vi "Lighthouse Monitoring & Control System 9.vi"() -> ()   [LabVIEW 2012]
uses:
  <vilib>/DAQmx/read.llb/DAQmx Read (Counter DBL 1Chan 1Samp).vi
  <vilib>/DAQmx/write.llb/DAQmx Write (Analog DBL 1Chan 1Samp).vi
  <vilib>/DAQmx/write.llb/DAQmx Write (Digital U8 1Chan 1Samp).vi
  <vilib>/DAQmx/write.llb/DAQmx Write (Digital 1D Bool NChan 1Samp 1Line).vi
  <vilib>/DAQmx/read.llb/DAQmx Read (Analog DBL 1Chan 1Samp).vi
  <vilib>/DAQmx/create/channels.llb/DAQmx Create Channel (CI-Count Edges).vi
  <vilib>/DAQmx/create/channels.llb/DAQmx Create Channel (DO-Digital Output).vi
  <vilib>/DAQmx/create/channels.llb/DAQmx Create Channel (AI-Voltage-Basic).vi
  <vilib>/DAQmx/create/channels.llb/DAQmx Create Channel (AO-Voltage-Basic).vi
  <vilib>/DAQmx/miscellaneous.llb/DAQmx Fill In Error Info.vi
panel:
  out "Time:":string
  out "Date:":string
  out "Voltage:":dbl
  out "Slot Count:":dbl
  in  "Dignostic Mode":bool
  in  "?":bool
  out "Data to Write":u32=255 caption="Data to Write:" format="%x"
  out "Motor:":bool[](array[boolean])
  out "3":bool
  out "2":bool
  out "1":bool
  # "Lighthouse Monitoring & Control System"
  # "Normal Mode"
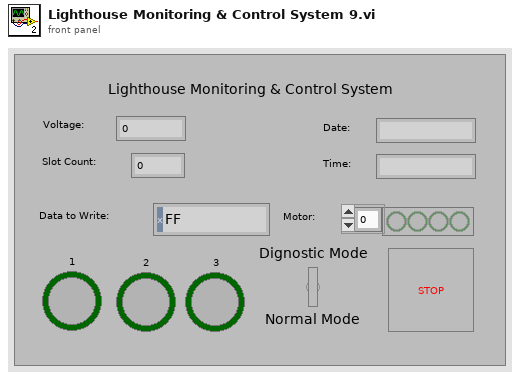
[diagram p1: front panel]
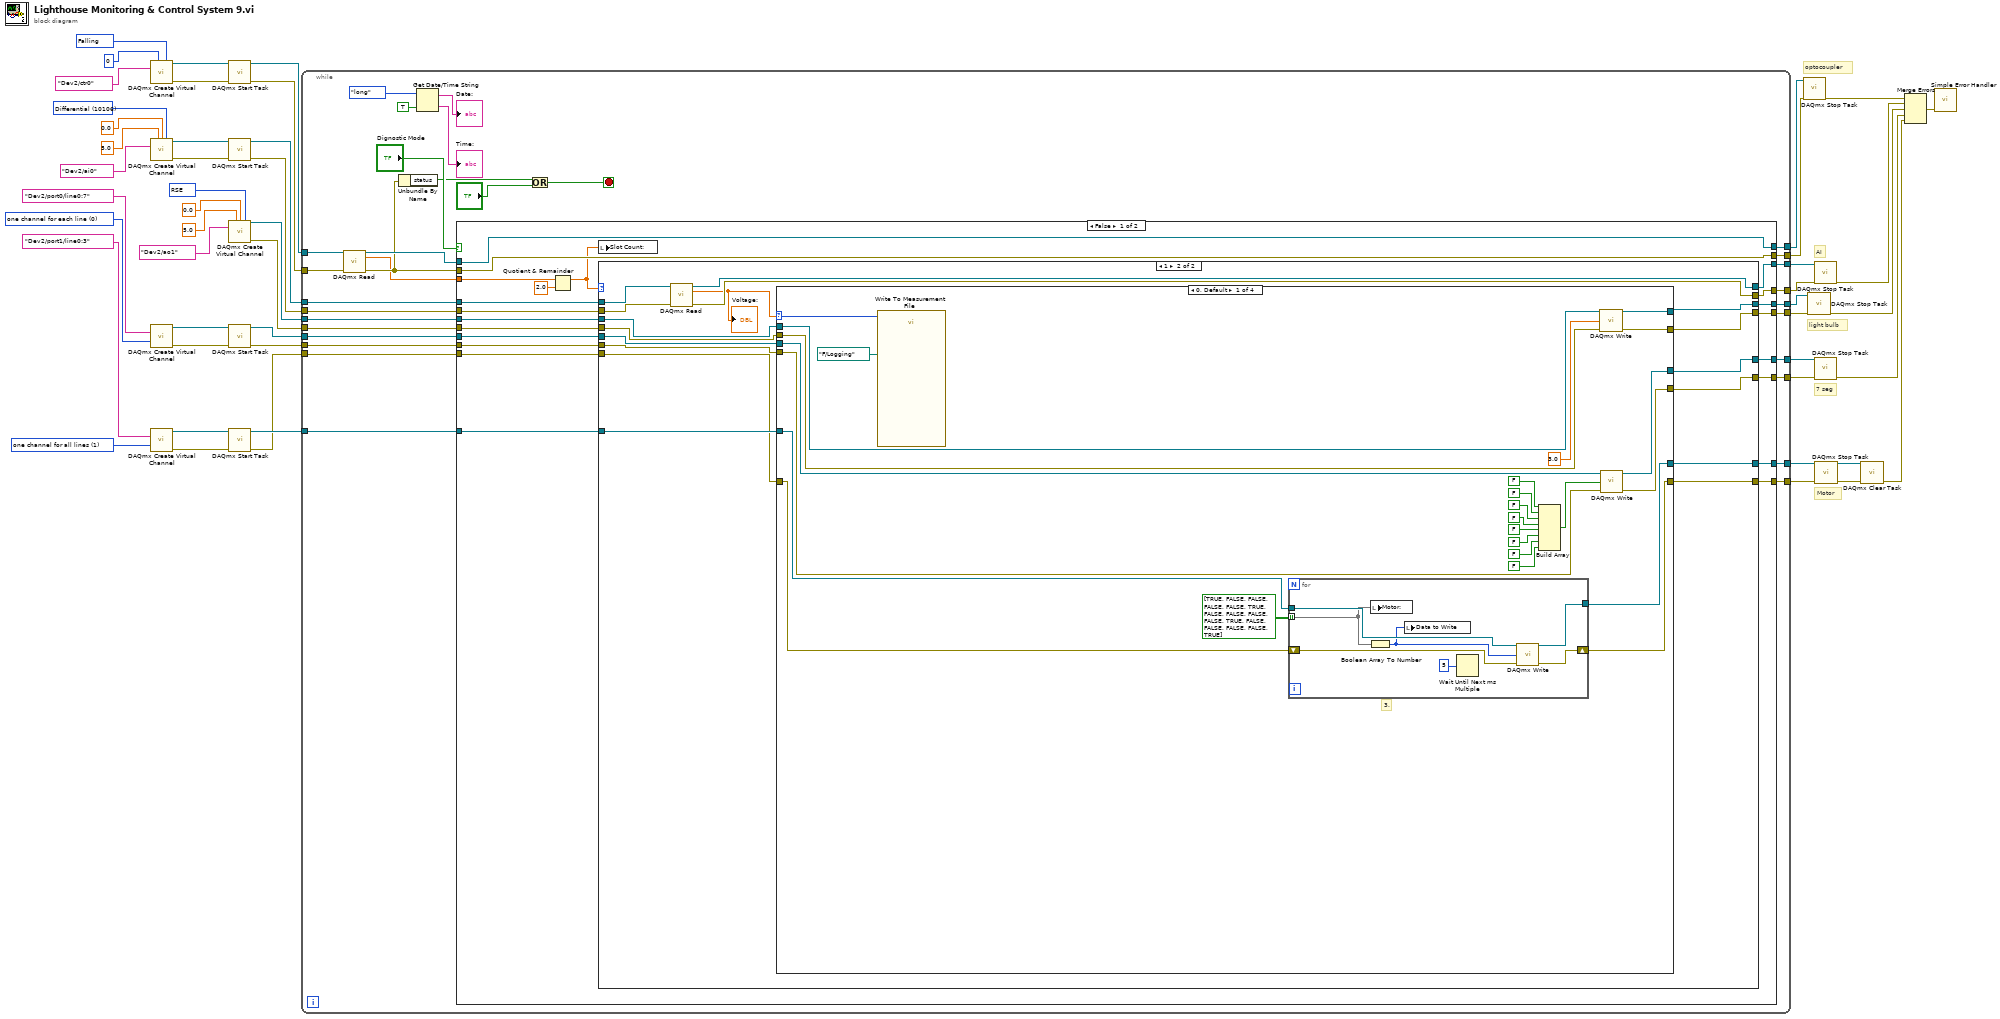
[diagram p0: block diagram]
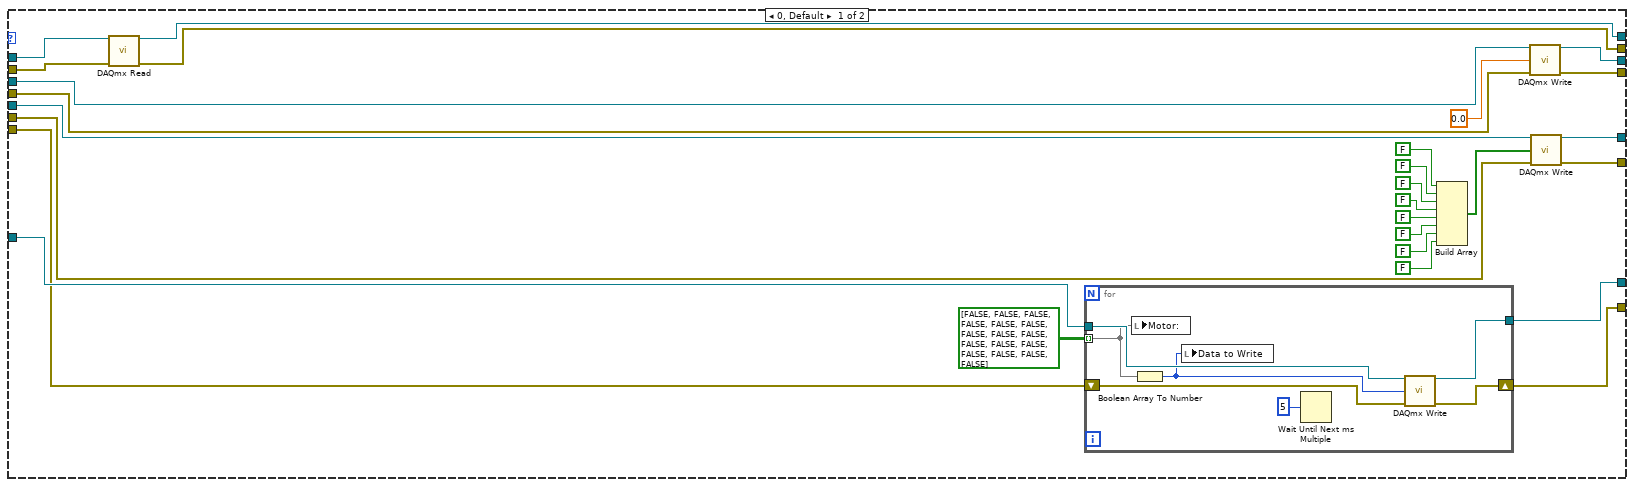
[diagram p2: hidden frame]
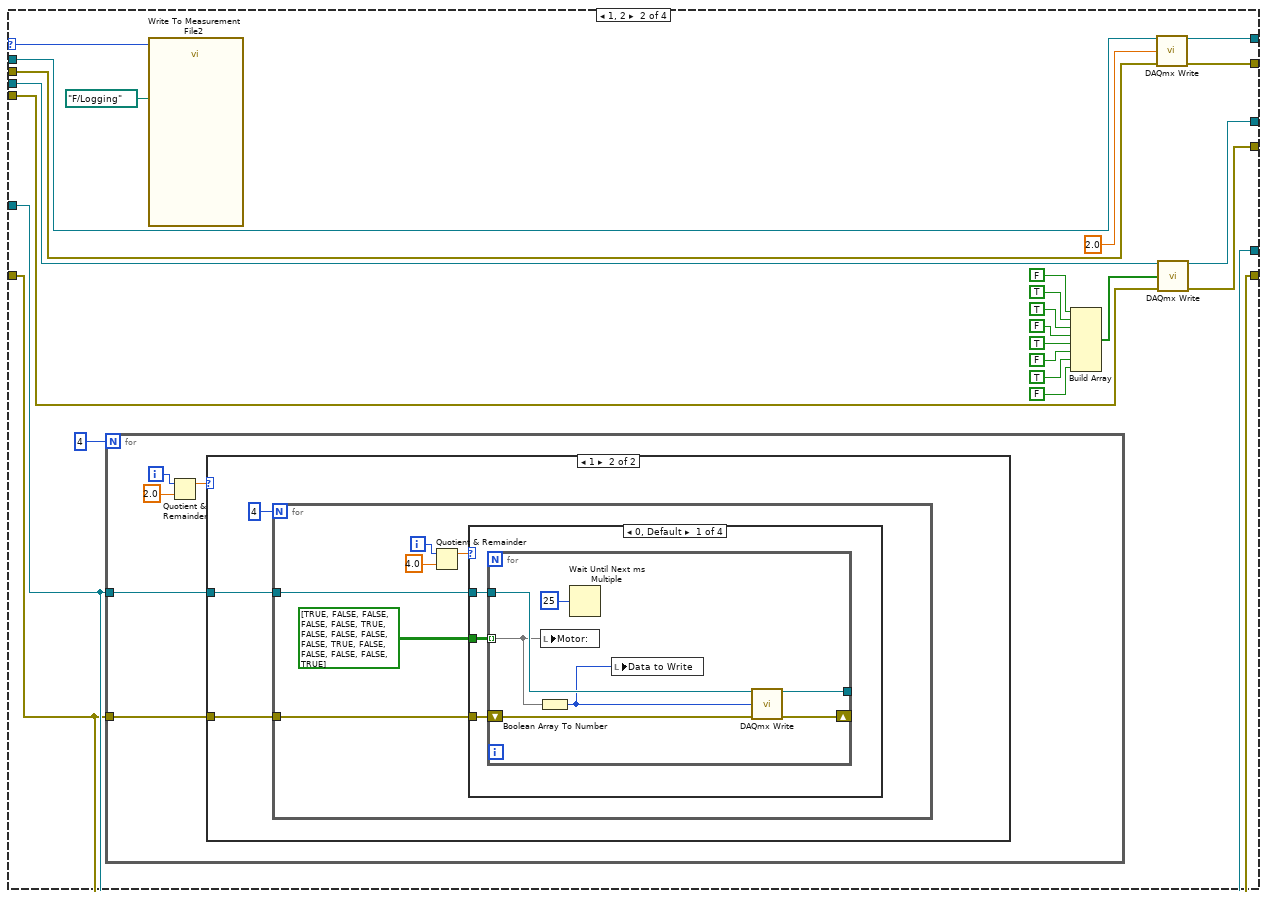
[diagram p3: hidden frame]
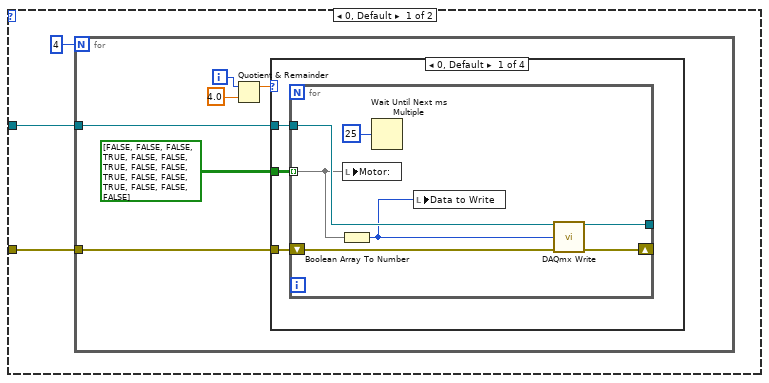
[diagram p4: hidden frame]
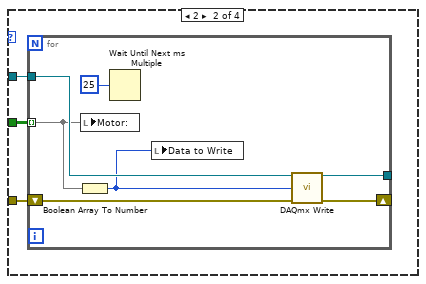
[diagram p5: hidden frame]
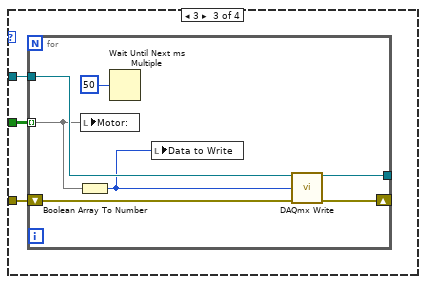
[diagram p6: hidden frame]
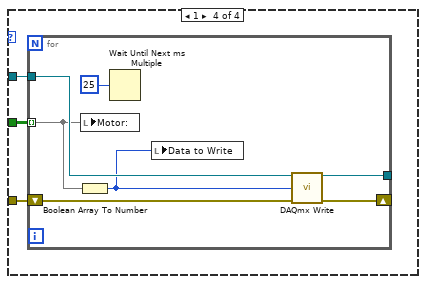
[diagram p7: hidden frame]
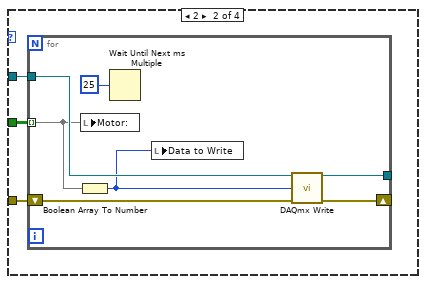
[diagram p8: hidden frame]
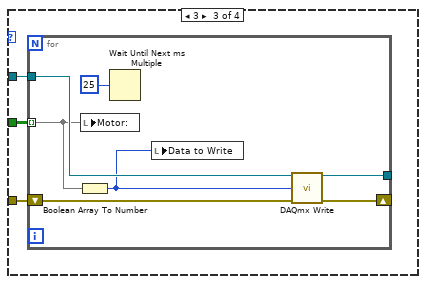
[diagram p9: hidden frame]
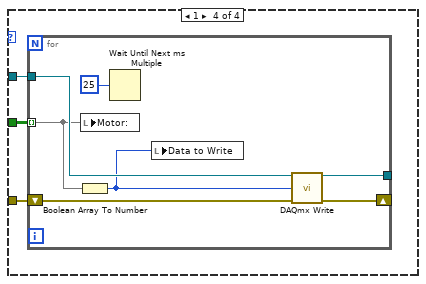
[diagram p10: hidden frame]
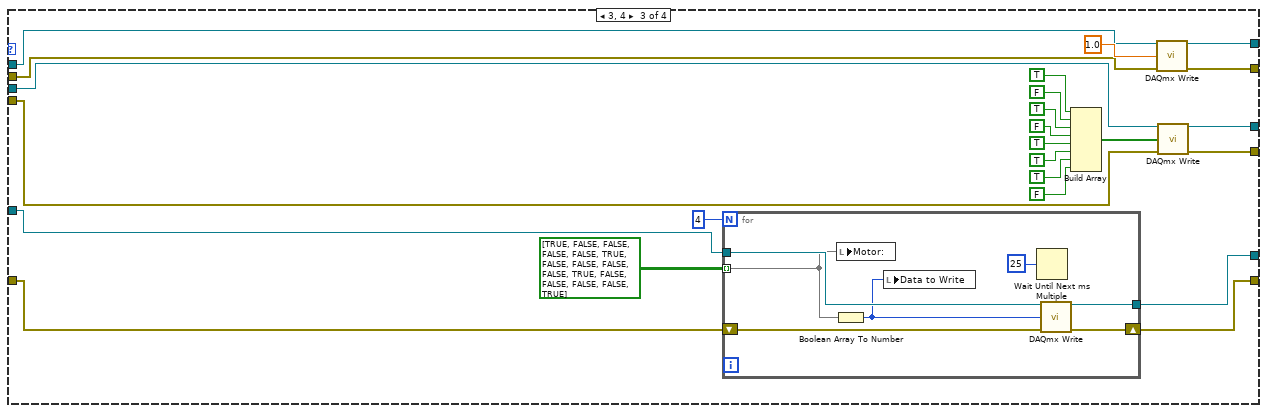
[diagram p11: hidden frame]
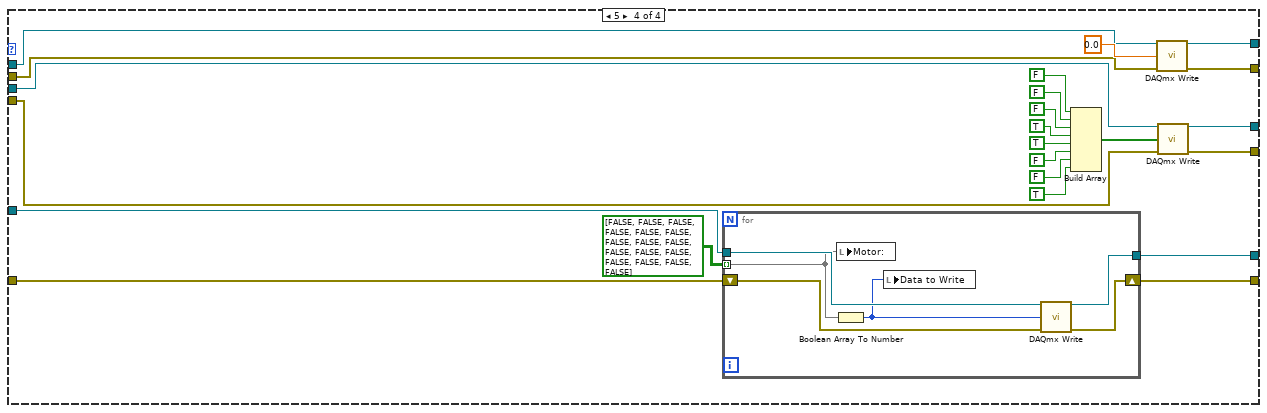
[diagram p12: hidden frame]
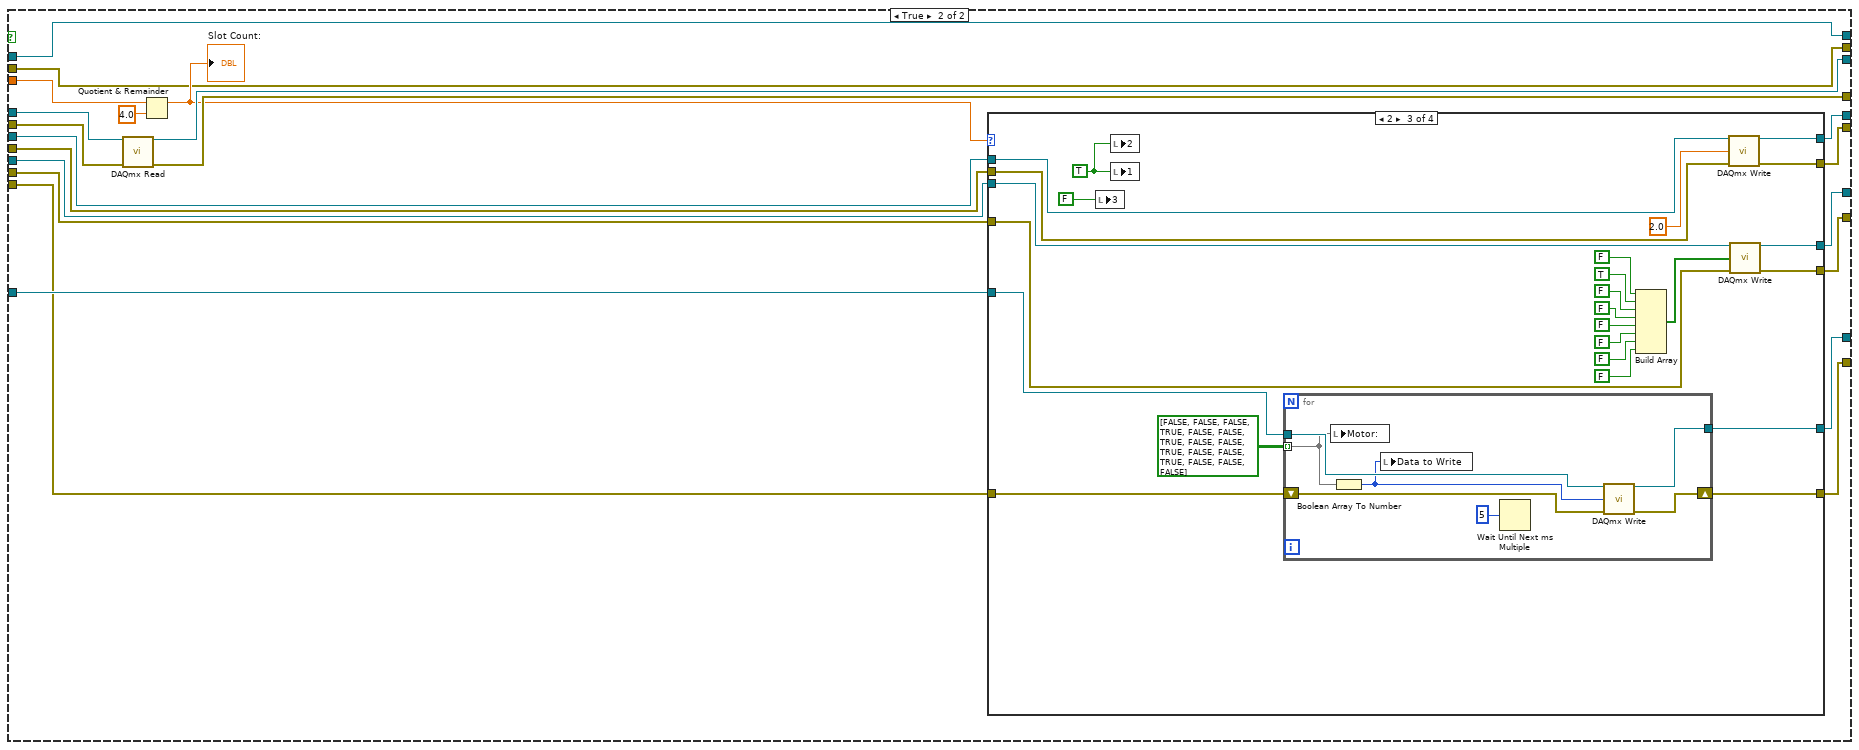
[diagram p13: hidden frame]
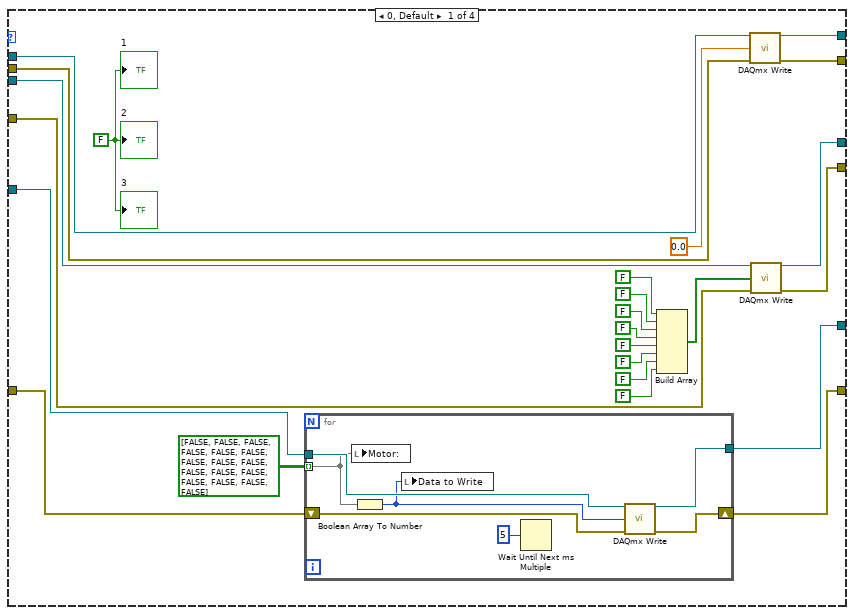
[diagram p14: hidden frame]
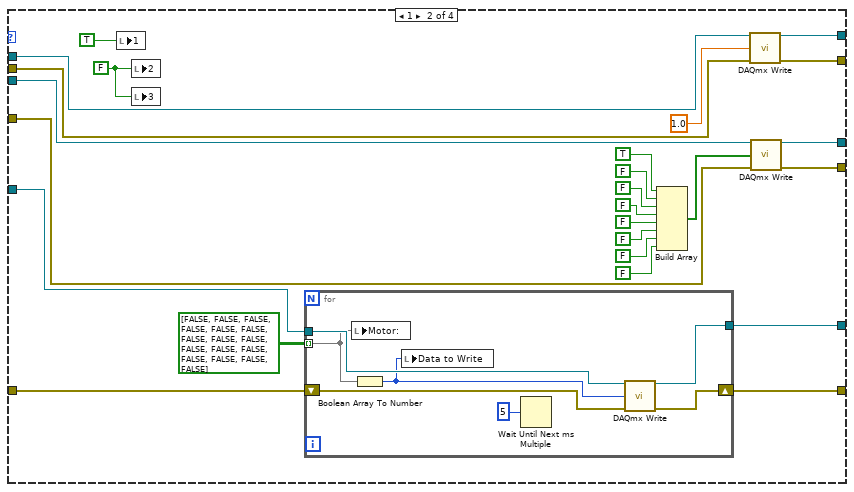
[diagram p15: hidden frame]
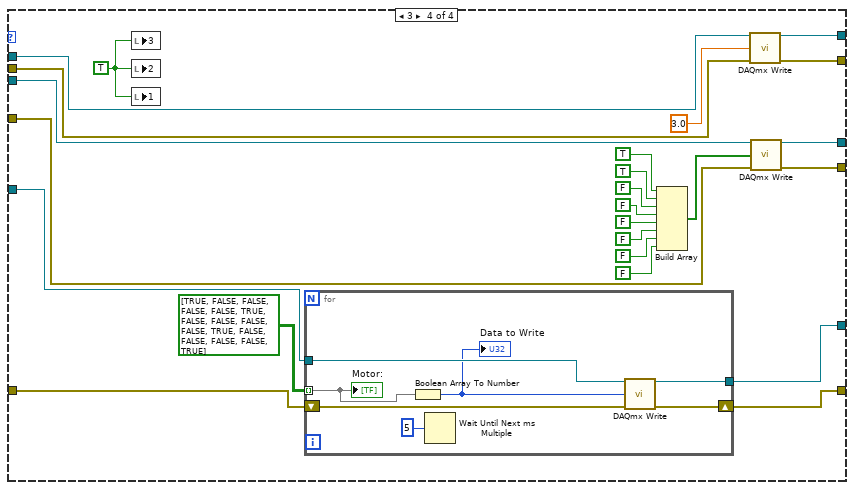
[diagram p16: hidden frame]
diagram:
  w24 = 10083 items=["Default"=-1, "RSE"=10083, "Differential"=10106, "Pseudodifferential"=12529] ("output terminal configuration")
  w32 = 10106 items=["default"=-1, "RSE"=10083, "NRSE"=10078, "Differential"=10106, "Pseudodifferential"=12529] ("input terminal configuration")
  w42 = 1 items=["one channel for each line", "one channel for all lines"] ("line grouping")
  w37 = 0 items=["one channel for each line", "one channel for all lines"] ("line grouping")
  w51 = 10171 items=["Rising"=10280, "Falling"=10171] ("edge")
  # "Motor"
  # "7 seg"
  # "AI"
  # "light bulb"
  # "optocoupler"
  n1 = call-poly <vilib>:"DAQmx Create Virtual Channel.vi"("initial count"=u32 0, "edge"=w51, "counter"=tag "Dev2/ctr0") -> ("task out"=w50:refnum<k21>, "error out"=w49:errorcluster)  [unwired: 11 in]
  n2 = call-poly <vilib>:"DAQmx Create Virtual Channel.vi"("maximum value"=5.0, "minimum value"=0.0, "input terminal configuration"=w32, "physical channels"=tag "Dev2/ai0") -> ("task out"=w30:refnum<k21>, "error out"=w31:errorcluster)  [unwired: 10 in]
  n3 = call-poly <vilib>:"DAQmx Create Virtual Channel.vi"("lines"=tag "Dev2/port0/line0:7", "line grouping"=w37) -> ("task out"=w44:refnum<k21>, "error out"=w43:errorcluster)  [unwired: 12 in]
  n4 = call-poly <vilib>:"DAQmx Create Virtual Channel.vi"("lines"=tag "Dev2/port1/line0:3", "line grouping"=w42) -> ("task out"=w41:refnum<k21>, "error out"=w40:errorcluster)  [unwired: 12 in]
  n5 = call <vilib>:"DAQmx Start Task.vi"("task/channels in"=w50, "error in"=w49) -> ("task out"=w46:refnum<k21>, "error out"=w45:errorcluster)  [unwired: 12 in]
  n6 = call <vilib>:"DAQmx Start Task.vi"("task/channels in"=w30, "error in"=w31) -> ("task out"=w26:refnum<k21>, "error out"=w25:errorcluster)  [unwired: 12 in]
  n7 = call-poly <vilib>:"DAQmx Create Virtual Channel.vi"("maximum value"=5.0, "minimum value"=0.0, "output terminal configuration"=w24, "physical channels"=tag "Dev2/ao1") -> ("task out"=w20:refnum<k21>, "error out"=w19:errorcluster)  [unwired: 10 in]
  n8 = call <vilib>:"DAQmx Start Task.vi"("task/channels in"=w44, "error in"=w43) -> ("task out"=w36:refnum<k21>, "error out"=w35:errorcluster)  [unwired: 12 in]
  n9 = call <vilib>:"DAQmx Start Task.vi"("task/channels in"=w41, "error in"=w40) -> ("task out"=w34:refnum<k21>, "error out"=w33:errorcluster)  [unwired: 12 in]
  n10 = while {
    tunnel: w46 -> [w81]
    tunnel: w45 -> [w80]
    tunnel: w36 -> [w79]
    tunnel: w35 -> [w78]
    tunnel: w34 -> [w77]
    tunnel: w33 -> [w76]
    tunnel: w26 -> [w74]
    tunnel: w25 -> [w73]
    tunnel: w20 -> [w72]
    tunnel: w19 -> [w71]
    tunnel: [w65] -> w10
    tunnel: [w64] -> w9
    tunnel: [w63] -> w8
    tunnel: [w62] -> w7
    tunnel: [w61] -> w6
    tunnel: [w60] -> w5
    tunnel: [w59] -> w4
    tunnel: [w58] -> w3
    tunnel: [w57] -> w2
    tunnel: [w56] -> w1
    stop <- w66 stop-if-true
    n11 = call-poly <vilib>:"DAQmx Read.vi"("task/channels in"=w81, "error in"=w80) -> ("task out"=w69:refnum<k21>, "data"=w67:dbl, "error out"=w68:errorcluster)  [unwired: 11 in]
    n12 = Unbundle By Name(w68) -> ("status"=w75:bool)
    n13 = Get Date/Time String(date format (0)=enum16{"short", "long", "abbreviated"}."long", want seconds? (F)=TRUE) -> (date string=→"Date:":string, time string=→"Time:":string)  [unwired: 1 in]
    n14 = case shown="False" "Dignostic Mode" {
      tunnel: w79 -> [w91 w393]
      tunnel: w78 -> [w90 w392]
      tunnel: w77 -> [w89 w391]
      tunnel: w76 -> [w88 w390]
      tunnel: [w87 w389] -> w59
      tunnel: [w86 w388] -> w58
      tunnel: w74 -> [w101 w385]
      tunnel: w73 -> [w100 w384]
      tunnel: w72 -> [w85 w387]
      tunnel: w71 -> [w84 w386]
      tunnel: [w99 w383] -> w57
      tunnel: [w98 w382] -> w56
      tunnel: [w97 w381] -> w63
      tunnel: [w96 w380] -> w62
      tunnel: [w93 w379] -> w60
      tunnel: [w92 w378] -> w61
      tunnel: w69 -> [w95 w374]
      tunnel: w68 -> [w94 w373]
      tunnel: w67 -> [w102 w376]
      tunnel: [w95 w374] -> w65
      tunnel: [w94 w373] -> w64
      frame False {
        n15 = Quotient & Remainder(x=w102, y=2.0) -> (x-y*floor(x/y)=w83:dbl)  [unwired: 1 out]
        n16 = local write "Slot Count:"(w83) -> ()
        n17 = case shown="1" w83 {
          tunnel: w101 -> [w129 w154]
          tunnel: w100 -> [w128 w153]
          tunnel: [w125 w152] -> w97
          tunnel: [w126 w151] -> w96
          tunnel: [w127 w150] -> w98
          tunnel: [w122 w149] -> w93
          tunnel: [w123 w148] -> w92
          tunnel: [w124 w147] -> w99
          tunnel: [w110 w145] -> w86
          tunnel: [w111 w146] -> w87
          tunnel: w91 -> [w109 w139]
          tunnel: w90 -> [w108 w138]
          tunnel: w89 -> [w107 w141]
          tunnel: w88 -> [w106 w140]
          tunnel: w85 -> [w105 w143]
          tunnel: w84 -> [w104 w142]
          frame 0, Default {
            n18 = call-poly <vilib>:"DAQmx Read.vi"("task/channels in"=w129, "error in"=w128) -> ("task out"=w124:refnum<k21>, "error out"=w127:errorcluster)  [unwired: 11 in, 1 out]
            n19 = for {
              tunnel: [w136] -> w111
              shift-right: [w134] -> w110
              shift-left: w106 -> [w137]
              tunnel: bool[][] [[FALSE, FALSE, FALSE, FALSE], [FALSE, FALSE, FALSE, FALSE], [FALSE, FALSE, FALSE, FALSE], [FALSE, FALSE, FALSE, FALSE]] -> [w131] mode=indexing
              tunnel: w107 -> [w133]
              n20 = local write "Motor:"(w131) -> ()
              n21 = Boolean Array To Number(Boolean array=w131) -> (number=w132:u32)
              n22 = local write "Data to Write"(w132) -> ()
              n23 = Wait Until Next ms Multiple(millisecond multiple=5) -> ()  [unwired: 1 out]
              n24 = call-poly <vilib>:"DAQmx Write.vi"("task/channels in"=w133, "data"=w132, "error in"=w137) -> ("task out"=w136:refnum<k21>, "error out"=w134:errorcluster)  [unwired: 10 in, 1 out]
            }
            n25 = Build Array(FALSE, FALSE, FALSE, FALSE, FALSE, FALSE, FALSE, FALSE) -> (w113:bool[])
            n26 = call-poly <vilib>:"DAQmx Write.vi"("task/channels in"=w105, "data"=0.0, "error in"=w104) -> ("task out"=w125:refnum<k21>, "error out"=w126:errorcluster)  [unwired: 10 in, 1 out]
            n27 = call-poly <vilib>:"DAQmx Write.vi"("task/channels in"=w109, "data"=w113, "error in"=w108) -> ("task out"=w123:refnum<k21>, "error out"=w122:errorcluster)  [unwired: 10 in, 1 out]
          }
          frame 1 {
            n28 = call-poly <vilib>:"DAQmx Read.vi"("task/channels in"=w154, "error in"=w153) -> ("task out"=w147:refnum<k21>, "data"=w144:dbl, "error out"=w150:errorcluster)  [unwired: 11 in]
            "Voltage:" <- w144
            n29 = case shown="0, Default" w144 {
              selector: w144 -> [w161 w194 _ _]
              tunnel: [w169 w199 w326 w356] -> w152
              tunnel: [w168 w198 w325 w355] -> w151
              tunnel: [w167 w197 w324 w354] -> w148
              tunnel: [w166 w196 w323 w353] -> w149
              tunnel: [w165 w188 w321 w351] -> w146
              tunnel: [w164 w187 w320 w350] -> w145
              tunnel: w143 -> [w160 w193 w319 w349]
              tunnel: w142 -> [w159 w192 w318 w348]
              tunnel: w141 -> [w158 w188 w315 w345]
              tunnel: w140 -> [w155 w187 w314 w344]
              tunnel: w139 -> [w157 w191 w317 w347]
              tunnel: w138 -> [w156 w190 w316 w346]
              frame 0, Default {
                # "3."
                n30 = call "Write To Measurement File"("Signals"=w161, "Filename"=path "F:/Logging") -> ()  [unwired: 15 in, 3 out]
                n31 = for {
                  tunnel: [w185] -> w165
                  shift-right: [w184] -> w164
                  shift-left: w155 -> [w186]
                  tunnel: bool[][] [[TRUE, FALSE, FALSE, FALSE], [FALSE, TRUE, FALSE, FALSE], [FALSE, FALSE, TRUE, FALSE], [FALSE, FALSE, FALSE, TRUE]] -> [w180] mode=indexing
                  tunnel: w158 -> [w182]
                  n32 = Boolean Array To Number(Boolean array=w180) -> (number=w181:u32)
                  n33 = local write "Motor:"(w180) -> ()
                  n34 = local write "Data to Write"(w181) -> ()
                  n35 = Wait Until Next ms Multiple(millisecond multiple=u32 5) -> ()  [unwired: 1 out]
                  n36 = call-poly <vilib>:"DAQmx Write.vi"("task/channels in"=w182, "data"=w181, "error in"=w186) -> ("task out"=w185:refnum<k21>, "error out"=w184:errorcluster)  [unwired: 10 in, 1 out]
                }
                n37 = Build Array(FALSE, FALSE, FALSE, FALSE, FALSE, FALSE, FALSE, FALSE) -> (w170:bool[])
                n38 = call-poly <vilib>:"DAQmx Write.vi"("task/channels in"=w160, "data"=3.0, "error in"=w159) -> ("task out"=w169:refnum<k21>, "error out"=w168:errorcluster)  [unwired: 10 in, 1 out]
                n39 = call-poly <vilib>:"DAQmx Write.vi"("task/channels in"=w157, "data"=w170, "error in"=w156) -> ("task out"=w167:refnum<k21>, "error out"=w166:errorcluster)  [unwired: 10 in, 1 out]
              }
              frame 1, 2 {
                n40 = for {
                  N: 4 -> [_]
                  tunnel: w188 -> [w214]
                  tunnel: w187 -> [w213]
                  i -> [w211]
                  n41 = Quotient & Remainder(x=w211, y=2.0) -> (x-y*floor(x/y)=w210:dbl)  [unwired: 1 out]
                  n42 = case shown="1" w210 {
                    tunnel: w214 -> [w217 w266]
                    tunnel: w213 -> [w216 w265]
                    frame 0, Default {
                      n43 = for {
                        N: 4 -> [_]
                        tunnel: w217 -> [w223]
                        tunnel: w216 -> [w222]
                        i -> [w219]
                        n44 = Quotient & Remainder(x=w219, y=4.0) -> (x-y*floor(x/y)=w218:dbl)  [unwired: 1 out]
                        n45 = case shown="0, Default" w218 {
                          tunnel: w223 -> [w226 w236 w245 w256]
                          tunnel: w222 -> [w224 w235 w246 w255]
                          tunnel: bool[][] [[FALSE, FALSE, FALSE, TRUE], [FALSE, FALSE, TRUE, FALSE], [FALSE, TRUE, FALSE, FALSE], [TRUE, FALSE, FALSE, FALSE]] -> [w225 w234 w244 w254]
                          frame 0, Default {
                            n46 = for {
                              tunnel: [w232] -> _
                              shift-right: [w231] -> _
                              shift-left: w224 -> [w233]
                              tunnel: w225 -> [w227] mode=indexing
                              tunnel: w226 -> [w229]
                              n47 = Boolean Array To Number(Boolean array=w227) -> (number=w228:u32)
                              n48 = local write "Motor:"(w227) -> ()
                              n49 = Wait Until Next ms Multiple(millisecond multiple=u32 25) -> ()  [unwired: 1 out]
                              n50 = local write "Data to Write"(w228) -> ()
                              n51 = call-poly <vilib>:"DAQmx Write.vi"("task/channels in"=w229, "data"=w228, "error in"=w233) -> ("task out"=w232:refnum<k21>, "error out"=w231:errorcluster)  [unwired: 10 in, 1 out]
                            }
                          }
                          frame 2 {
                            n52 = for {
                              tunnel: [w242] -> _
                              shift-right: [w241] -> _
                              shift-left: w235 -> [w243]
                              tunnel: w234 -> [w237] mode=indexing
                              tunnel: w236 -> [w239]
                              n53 = Boolean Array To Number(Boolean array=w237) -> (number=w238:u32)
                              n54 = local write "Motor:"(w237) -> ()
                              n55 = Wait Until Next ms Multiple(millisecond multiple=u32 25) -> ()  [unwired: 1 out]
                              n56 = local write "Data to Write"(w238) -> ()
                              n57 = call-poly <vilib>:"DAQmx Write.vi"("task/channels in"=w239, "data"=w238, "error in"=w243) -> ("task out"=w242:refnum<k21>, "error out"=w241:errorcluster)  [unwired: 10 in, 1 out]
                            }
                          }
                          frame 3 {
                            n58 = for {
                              tunnel: [w252] -> _
                              shift-right: [w251] -> _
                              shift-left: w246 -> [w253]
                              tunnel: w244 -> [w248] mode=indexing
                              tunnel: w245 -> [w249]
                              n59 = Boolean Array To Number(Boolean array=w248) -> (number=w247:u32)
                              n60 = local write "Motor:"(w248) -> ()
                              n61 = Wait Until Next ms Multiple(millisecond multiple=u32 50) -> ()  [unwired: 1 out]
                              n62 = local write "Data to Write"(w247) -> ()
                              n63 = call-poly <vilib>:"DAQmx Write.vi"("task/channels in"=w249, "data"=w247, "error in"=w253) -> ("task out"=w252:refnum<k21>, "error out"=w251:errorcluster)  [unwired: 10 in, 1 out]
                            }
                          }
                          frame 1 {
                            n64 = for {
                              tunnel: [w262] -> _
                              shift-right: [w261] -> _
                              shift-left: w255 -> [w263]
                              tunnel: w254 -> [w258] mode=indexing
                              tunnel: w256 -> [w259]
                              n65 = Boolean Array To Number(Boolean array=w258) -> (number=w257:u32)
                              n66 = local write "Motor:"(w258) -> ()
                              n67 = Wait Until Next ms Multiple(millisecond multiple=u32 25) -> ()  [unwired: 1 out]
                              n68 = local write "Data to Write"(w257) -> ()
                              n69 = call-poly <vilib>:"DAQmx Write.vi"("task/channels in"=w259, "data"=w257, "error in"=w263) -> ("task out"=w262:refnum<k21>, "error out"=w261:errorcluster)  [unwired: 10 in, 1 out]
                            }
                          }
                        }
                      }
                    }
                    frame 1 {
                      n70 = for {
                        N: 4 -> [_]
                        tunnel: w266 -> [w272]
                        tunnel: w265 -> [w271]
                        i -> [w270]
                        n71 = Quotient & Remainder(x=w270, y=4.0) -> (x-y*floor(x/y)=w268:dbl)  [unwired: 1 out]
                        n72 = case shown="0, Default" w268 {
                          tunnel: w272 -> [w275 w285 w294 w305]
                          tunnel: w271 -> [w274 w284 w295 w304]
                          tunnel: bool[][] [[TRUE, FALSE, FALSE, FALSE], [FALSE, TRUE, FALSE, FALSE], [FALSE, FALSE, TRUE, FALSE], [FALSE, FALSE, FALSE, TRUE]] -> [w273 w283 w293 w303]
                          frame 0, Default {
                            n73 = for {
                              tunnel: [w281] -> _
                              shift-right: [w280] -> _
                              shift-left: w274 -> [w282]
                              tunnel: w273 -> [w277] mode=indexing
                              tunnel: w275 -> [w278]
                              n74 = Boolean Array To Number(Boolean array=w277) -> (number=w276:u32)
                              n75 = local write "Motor:"(w277) -> ()
                              n76 = Wait Until Next ms Multiple(millisecond multiple=u32 25) -> ()  [unwired: 1 out]
                              n77 = local write "Data to Write"(w276) -> ()
                              n78 = call-poly <vilib>:"DAQmx Write.vi"("task/channels in"=w278, "data"=w276, "error in"=w282) -> ("task out"=w281:refnum<k21>, "error out"=w280:errorcluster)  [unwired: 10 in, 1 out]
                            }
                          }
                          frame 2 {
                            n79 = for {
                              tunnel: [w291] -> _
                              shift-right: [w290] -> _
                              shift-left: w284 -> [w292]
                              tunnel: w283 -> [w286] mode=indexing
                              tunnel: w285 -> [w288]
                              n80 = Boolean Array To Number(Boolean array=w286) -> (number=w287:u32)
                              n81 = local write "Motor:"(w286) -> ()
                              n82 = Wait Until Next ms Multiple(millisecond multiple=u32 25) -> ()  [unwired: 1 out]
                              n83 = local write "Data to Write"(w287) -> ()
                              n84 = call-poly <vilib>:"DAQmx Write.vi"("task/channels in"=w288, "data"=w287, "error in"=w292) -> ("task out"=w291:refnum<k21>, "error out"=w290:errorcluster)  [unwired: 10 in, 1 out]
                            }
                          }
                          frame 3 {
                            n85 = for {
                              tunnel: [w301] -> _
                              shift-right: [w300] -> _
                              shift-left: w295 -> [w302]
                              tunnel: w293 -> [w297] mode=indexing
                              tunnel: w294 -> [w298]
                              n86 = Boolean Array To Number(Boolean array=w297) -> (number=w296:u32)
                              n87 = local write "Motor:"(w297) -> ()
                              n88 = Wait Until Next ms Multiple(millisecond multiple=u32 25) -> ()  [unwired: 1 out]
                              n89 = local write "Data to Write"(w296) -> ()
                              n90 = call-poly <vilib>:"DAQmx Write.vi"("task/channels in"=w298, "data"=w296, "error in"=w302) -> ("task out"=w301:refnum<k21>, "error out"=w300:errorcluster)  [unwired: 10 in, 1 out]
                            }
                          }
                          frame 1 {
                            n91 = for {
                              tunnel: [w311] -> _
                              shift-right: [w310] -> _
                              shift-left: w304 -> [w312]
                              tunnel: w303 -> [w307] mode=indexing
                              tunnel: w305 -> [w308]
                              n92 = Boolean Array To Number(Boolean array=w307) -> (number=w306:u32)
                              n93 = local write "Motor:"(w307) -> ()
                              n94 = Wait Until Next ms Multiple(millisecond multiple=u32 25) -> ()  [unwired: 1 out]
                              n95 = local write "Data to Write"(w306) -> ()
                              n96 = call-poly <vilib>:"DAQmx Write.vi"("task/channels in"=w308, "data"=w306, "error in"=w312) -> ("task out"=w311:refnum<k21>, "error out"=w310:errorcluster)  [unwired: 10 in, 1 out]
                            }
                          }
                        }
                      }
                    }
                  }
                }
                n97 = call "Write To Measurement File2"("Signals"=w194, "Filename"=path "F:/Logging") -> ()  [unwired: 15 in, 3 out]
                n98 = Build Array(FALSE, TRUE, TRUE, FALSE, TRUE, FALSE, TRUE, FALSE) -> (w200:bool[])
                n99 = call-poly <vilib>:"DAQmx Write.vi"("task/channels in"=w193, "data"=2.0, "error in"=w192) -> ("task out"=w199:refnum<k21>, "error out"=w198:errorcluster)  [unwired: 10 in, 1 out]
                n100 = call-poly <vilib>:"DAQmx Write.vi"("task/channels in"=w191, "data"=w200, "error in"=w190) -> ("task out"=w197:refnum<k21>, "error out"=w196:errorcluster)  [unwired: 10 in, 1 out]
              }
              frame 3, 4 {
                n101 = for {
                  N: 4 -> [_]
                  tunnel: [w342] -> w321
                  shift-right: [w341] -> w320
                  shift-left: w314 -> [w343]
                  tunnel: bool[][] [[TRUE, FALSE, FALSE, FALSE], [FALSE, TRUE, FALSE, FALSE], [FALSE, FALSE, TRUE, FALSE], [FALSE, FALSE, FALSE, TRUE]] -> [w338] mode=indexing
                  tunnel: w315 -> [w340]
                  n102 = Boolean Array To Number(Boolean array=w338) -> (number=w339:u32)
                  n103 = local write "Motor:"(w338) -> ()
                  n104 = local write "Data to Write"(w339) -> ()
                  n105 = Wait Until Next ms Multiple(millisecond multiple=u32 25) -> ()  [unwired: 1 out]
                  n106 = call-poly <vilib>:"DAQmx Write.vi"("task/channels in"=w340, "data"=w339, "error in"=w343) -> ("task out"=w342:refnum<k21>, "error out"=w341:errorcluster)  [unwired: 10 in, 1 out]
                }
                n107 = Build Array(TRUE, FALSE, TRUE, FALSE, TRUE, TRUE, TRUE, FALSE) -> (w327:bool[])
                n108 = call-poly <vilib>:"DAQmx Write.vi"("task/channels in"=w319, "data"=1.0, "error in"=w318) -> ("task out"=w326:refnum<k21>, "error out"=w325:errorcluster)  [unwired: 10 in, 1 out]
                n109 = call-poly <vilib>:"DAQmx Write.vi"("task/channels in"=w317, "data"=w327, "error in"=w316) -> ("task out"=w324:refnum<k21>, "error out"=w323:errorcluster)  [unwired: 10 in, 1 out]
              }
              frame 5 {
                n110 = for {
                  tunnel: [w371] -> w351
                  shift-right: [w370] -> w350
                  shift-left: w344 -> [w372]
                  tunnel: bool[][] [[FALSE, FALSE, FALSE, FALSE], [FALSE, FALSE, FALSE, FALSE], [FALSE, FALSE, FALSE, FALSE], [FALSE, FALSE, FALSE, FALSE]] -> [w367] mode=indexing
                  tunnel: w345 -> [w369]
                  n111 = Boolean Array To Number(Boolean array=w367) -> (number=w368:u32)
                  n112 = local write "Motor:"(w367) -> ()
                  n113 = local write "Data to Write"(w368) -> ()
                  n114 = call-poly <vilib>:"DAQmx Write.vi"("task/channels in"=w369, "data"=w368, "error in"=w372) -> ("task out"=w371:refnum<k21>, "error out"=w370:errorcluster)  [unwired: 10 in, 1 out]
                }
                n115 = Build Array(FALSE, FALSE, FALSE, TRUE, TRUE, FALSE, FALSE, TRUE) -> (w357:bool[])
                n116 = call-poly <vilib>:"DAQmx Write.vi"("task/channels in"=w349, "data"=0.0, "error in"=w348) -> ("task out"=w356:refnum<k21>, "error out"=w355:errorcluster)  [unwired: 10 in, 1 out]
                n117 = call-poly <vilib>:"DAQmx Write.vi"("task/channels in"=w347, "data"=w357, "error in"=w346) -> ("task out"=w354:refnum<k21>, "error out"=w353:errorcluster)  [unwired: 10 in, 1 out]
              }
            }
          }
        }
      }
      frame True {
        n118 = call-poly <vilib>:"DAQmx Read.vi"("task/channels in"=w385, "error in"=w384) -> ("task out"=w383:refnum<k21>, "error out"=w382:errorcluster)  [unwired: 11 in, 1 out]
        n119 = Quotient & Remainder(x=w376, y=4.0) -> (x-y*floor(x/y)=w375:dbl)  [unwired: 1 out]
        "Slot Count:" <- w375
        n120 = case shown="2" w375 {
          tunnel: w393 -> [w405 w433 w465 w496]
          tunnel: w392 -> [w404 w432 w466 w497]
          tunnel: w391 -> [w417 w431 w462 w494]
          tunnel: w390 -> [w416 w430 w463 w493]
          tunnel: [w415 w429 w461 w492] -> w389
          tunnel: [w414 w428 w460 w491] -> w388
          tunnel: w387 -> [w402 w444 w478 w509]
          tunnel: w386 -> [w401 w443 w477 w508]
          tunnel: [w400 w446 w480 w511] -> w381
          tunnel: [w399 w445 w479 w510] -> w380
          tunnel: [w396 w426 w458 w490] -> w378
          tunnel: [w395 w425 w457 w489] -> w379
          frame 0, Default {
            w397 = FALSE
            n121 = for {
              tunnel: [w423] -> w415
              shift-right: [w421] -> w414
              shift-left: w416 -> [w424]
              tunnel: w417 -> [w420]
              tunnel: bool[][] [[FALSE, FALSE, FALSE, FALSE], [FALSE, FALSE, FALSE, FALSE], [FALSE, FALSE, FALSE, FALSE], [FALSE, FALSE, FALSE, FALSE]] -> [w418] mode=indexing
              n122 = local write "Motor:"(w418) -> ()
              n123 = Boolean Array To Number(Boolean array=w418) -> (number=w419:u32)
              n124 = local write "Data to Write"(w419) -> ()
              n125 = Wait Until Next ms Multiple(millisecond multiple=5) -> ()  [unwired: 1 out]
              n126 = call-poly <vilib>:"DAQmx Write.vi"("task/channels in"=w420, "data"=w419, "error in"=w424) -> ("task out"=w423:refnum<k21>, "error out"=w421:errorcluster)  [unwired: 10 in, 1 out]
            }
            n127 = Build Array(FALSE, FALSE, FALSE, FALSE, FALSE, FALSE, FALSE, FALSE) -> (w406:bool[])
            n128 = call-poly <vilib>:"DAQmx Write.vi"("task/channels in"=w402, "data"=0.0, "error in"=w401) -> ("task out"=w400:refnum<k21>, "error out"=w399:errorcluster)  [unwired: 10 in, 1 out]
            n129 = call-poly <vilib>:"DAQmx Write.vi"("task/channels in"=w405, "data"=w406, "error in"=w404) -> ("task out"=w396:refnum<k21>, "error out"=w395:errorcluster)  [unwired: 10 in, 1 out]
            "1" <- w397
            "2" <- w397
            "3" <- w397
          }
          frame 1 {
            w449 = FALSE ("LED 2")
            n130 = local write "1"(TRUE ("LED 1")) -> ()
            n131 = local write "2"(w449) -> ()
            n132 = local write "3"(w449) -> ()
            n133 = for {
              tunnel: [w455] -> w429
              shift-right: [w453] -> w428
              shift-left: w430 -> [w456]
              tunnel: w431 -> [w452]
              tunnel: bool[][] [[FALSE, FALSE, FALSE, FALSE], [FALSE, FALSE, FALSE, FALSE], [FALSE, FALSE, FALSE, FALSE], [FALSE, FALSE, FALSE, FALSE]] -> [w451] mode=indexing
              n134 = local write "Motor:"(w451) -> ()
              n135 = Boolean Array To Number(Boolean array=w451) -> (number=w450:u32)
              n136 = local write "Data to Write"(w450) -> ()
              n137 = Wait Until Next ms Multiple(millisecond multiple=5) -> ()  [unwired: 1 out]
              n138 = call-poly <vilib>:"DAQmx Write.vi"("task/channels in"=w452, "data"=w450, "error in"=w456) -> ("task out"=w455:refnum<k21>, "error out"=w453:errorcluster)  [unwired: 10 in, 1 out]
            }
            n139 = Build Array(TRUE, FALSE, FALSE, FALSE, FALSE, FALSE, FALSE, FALSE) -> (w434:bool[])
            n140 = call-poly <vilib>:"DAQmx Write.vi"("task/channels in"=w444, "data"=1.0, "error in"=w443) -> ("task out"=w446:refnum<k21>, "error out"=w445:errorcluster)  [unwired: 10 in, 1 out]
            n141 = call-poly <vilib>:"DAQmx Write.vi"("task/channels in"=w433, "data"=w434, "error in"=w432) -> ("task out"=w426:refnum<k21>, "error out"=w425:errorcluster)  [unwired: 10 in, 1 out]
          }
          frame 2 {
            w476 = TRUE ("LED 2")
            n142 = local write "3"(FALSE ("LED 3")) -> ()
            n143 = local write "2"(w476) -> ()
            n144 = local write "1"(w476) -> ()
            n145 = for {
              tunnel: [w487] -> w461
              shift-right: [w485] -> w460
              shift-left: w463 -> [w488]
              tunnel: w462 -> [w484]
              tunnel: bool[][] [[FALSE, FALSE, FALSE, TRUE], [FALSE, FALSE, TRUE, FALSE], [FALSE, TRUE, FALSE, FALSE], [TRUE, FALSE, FALSE, FALSE]] -> [w482] mode=indexing
              n146 = local write "Motor:"(w482) -> ()
              n147 = Boolean Array To Number(Boolean array=w482) -> (number=w483:u32)
              n148 = local write "Data to Write"(w483) -> ()
              n149 = Wait Until Next ms Multiple(millisecond multiple=5) -> ()  [unwired: 1 out]
              n150 = call-poly <vilib>:"DAQmx Write.vi"("task/channels in"=w484, "data"=w483, "error in"=w488) -> ("task out"=w487:refnum<k21>, "error out"=w485:errorcluster)  [unwired: 10 in, 1 out]
            }
            n151 = Build Array(FALSE ("element"), TRUE, FALSE, FALSE, FALSE, FALSE, FALSE, FALSE) -> (w467:bool[])
            n152 = call-poly <vilib>:"DAQmx Write.vi"("task/channels in"=w478, "data"=2.0, "error in"=w477) -> ("task out"=w480:refnum<k21>, "error out"=w479:errorcluster)  [unwired: 10 in, 1 out]
            n153 = call-poly <vilib>:"DAQmx Write.vi"("task/channels in"=w465, "data"=w467, "error in"=w466) -> ("task out"=w458:refnum<k21>, "error out"=w457:errorcluster)  [unwired: 10 in, 1 out]
          }
          frame 3 {
            w507 = TRUE ("LED 3")
            n154 = local write "3"(w507) -> ()
            n155 = local write "2"(w507) -> ()
            n156 = local write "1"(w507) -> ()
            n157 = for {
              tunnel: [w518] -> w492
              shift-right: [w516] -> w491
              shift-left: w493 -> [w519]
              tunnel: w494 -> [w515]
              tunnel: bool[][] [[TRUE, FALSE, FALSE, FALSE], [FALSE, TRUE, FALSE, FALSE], [FALSE, FALSE, TRUE, FALSE], [FALSE, FALSE, FALSE, TRUE]] -> [w513] mode=indexing
              n158 = Boolean Array To Number(Boolean array=w513) -> (number=w514:u32)
              "Data to Write" <- w514
              n159 = Wait Until Next ms Multiple(millisecond multiple=5) -> ()  [unwired: 1 out]
              n160 = call-poly <vilib>:"DAQmx Write.vi"("task/channels in"=w515, "data"=w514, "error in"=w519) -> ("task out"=w518:refnum<k21>, "error out"=w516:errorcluster)  [unwired: 10 in, 1 out]
              "Motor:" <- w513
            }
            n161 = Build Array(TRUE, TRUE, FALSE, FALSE, FALSE, FALSE, FALSE, FALSE) -> (w498:bool[])
            n162 = call-poly <vilib>:"DAQmx Write.vi"("task/channels in"=w509, "data"=3.0, "error in"=w508) -> ("task out"=w511:refnum<k21>, "error out"=w510:errorcluster)  [unwired: 10 in, 1 out]
            n163 = call-poly <vilib>:"DAQmx Write.vi"("task/channels in"=w496, "data"=w498, "error in"=w497) -> ("task out"=w490:refnum<k21>, "error out"=w489:errorcluster)  [unwired: 10 in, 1 out]
          }
        }
      }
    }
    n164 = Or(x=w75, y="?") -> (x .or. y?=w66:bool)
  }
  n165 = call <vilib>:"DAQmx Stop Task.vi"("task/channels in"=w10, "error in"=w9) -> ("error out"=w18:errorcluster)  [unwired: 12 in, 1 out]
  n166 = call <vilib>:"DAQmx Stop Task.vi"("task/channels in"=w8, "error in"=w7) -> ("error out"=w16:errorcluster)  [unwired: 12 in, 1 out]
  n167 = call <vilib>:"DAQmx Stop Task.vi"("task/channels in"=w2, "error in"=w1) -> ("error out"=w17:errorcluster)  [unwired: 12 in, 1 out]
  n168 = call <vilib>:"DAQmx Stop Task.vi"("task/channels in"=w6, "error in"=w5) -> ("error out"=w15:errorcluster)  [unwired: 12 in, 1 out]
  n169 = call <vilib>:"DAQmx Stop Task.vi"("task/channels in"=w4, "error in"=w3) -> ("task out"=w13:refnum<k21>, "error out"=w12:errorcluster)  [unwired: 12 in]
  n170 = call <vilib>:"DAQmx Clear Task.vi"("task in"=w13, "error in"=w12) -> ("error out"=w11:errorcluster)  [unwired: 13 in]
  n171 = Merge Errors(w18, w17, w16, w15, w11) -> (w14:errorcluster)
  n172 = call <vilib>:"Simple Error Handler.vi"("error in (no error)"=w14) -> ()  [unwired: 4 in, 5 out]
